vi "Scorer.vi"(8 "error in (no error)":errorcluster, 10 "Guess":i32, 11 "Answer":i32) -> (0 "error out":errorcluster, 1 "Minuses":i32, 2 "Pluses":i32, 3 "Result":string)   [LabVIEW 2017]
doc: "This VI takes two valid number inputs, the correct <b>Answer</b> and the player's <b>Guess</b>. \nIt produces a string <b>Result</b> and two numeric outputs describing the score."
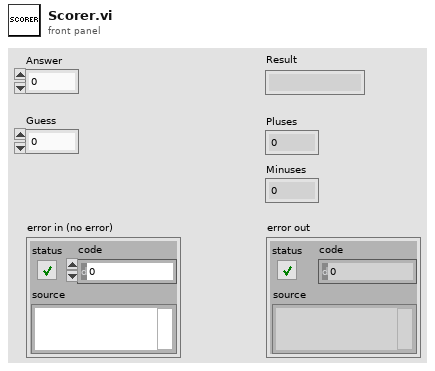
[diagram p1: front panel]
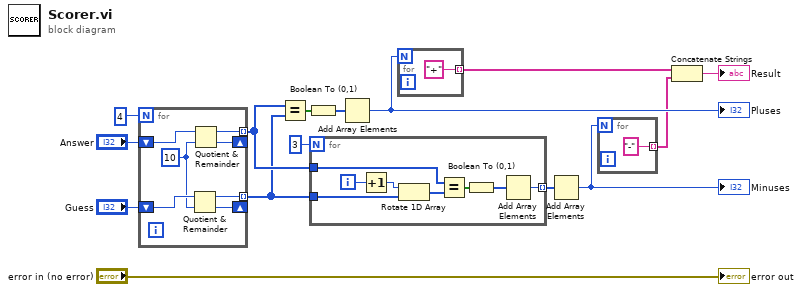
[diagram p0: block diagram]
diagram:
  n1 = for {
    N: 4 -> [_]
    shift-right: [w19] -> _
    shift-left: "Answer" -> [w22]
    shift-right: [w20] -> _
    shift-left: "Guess" -> [w21]
    tunnel: [w18] -> w10 mode=indexing
    tunnel: [w17] -> w9 mode=indexing
    w16 = 10
    n2 = Quotient & Remainder(x=w21, y=w16) -> (x-y*floor(x/y)=w17:i32, floor(x/y)=w20:i32)
    n3 = Quotient & Remainder(x=w22, y=w16) -> (x-y*floor(x/y)=w18:i32, floor(x/y)=w19:i32)
  }
  n4 = Equal?(x=w10, y=w9) -> (x = y?=w12:bool[])
  n5 = Boolean To (0,1)(Boolean=w12) -> (0, 1=w11:i16[])
  n6 = for {
    N: 3 -> [_]
    tunnel: w10 -> [w26]
    tunnel: w9 -> [w30]
    tunnel: [w23] -> w8 mode=indexing
    i -> [w29]
    n7 = Increment(x=w29) -> (x+1=w28:i32)
    n8 = Rotate 1D Array(1:w30, 2:w28) -> (0:w27:i32[])
    n9 = Equal?(x=w26, y=w27) -> (x = y?=w24:bool[])
    n10 = Boolean To (0,1)(Boolean=w24) -> (0, 1=w25:i16[])
    n11 = Add Array Elements(numeric array=w25) -> (sum=w23:i16)
  }
  n12 = Add Array Elements(numeric array=w11) -> (sum=w6:i16)
  "Pluses" <- w6
  n13 = for {
    N: w6 -> [_]
    tunnel: ["+"] -> w4 mode=indexing
  }
  n14 = Add Array Elements(numeric array=w8) -> (sum=w5:i16)
  "Minuses" <- w5
  n15 = for {
    N: w5 -> [_]
    tunnel: ["-"] -> w3 mode=indexing
  }
  n16 = Concatenate Strings(w4, w3) -> (→"Result":string)
  "error out" <- "error in (no error)"
